vi "If Error, then NaN.vi"(5 "clear error (F)":bool, 6 "error in (T)":errorcluster={"status"=TRUE, "code"=-1, "source"="If Error, then NaN.vi"}, 7 "value3":dbl=3.0, 8 "value2":dbl=2.0, 9 "value1":dbl=1.0) -> (0 "error out":errorcluster, 1 "value out3":dbl=nan, 2 "value out2":dbl=nan, 3 "value out1":dbl=nan)   [LabVIEW 2020]
doc: "This function enables an error to be ignored, but marked with a NaN value in a double precision floating point variable.\n\nIf \"error in\" is TRUE, then \"value out\" is set to NaN, else \"value out\" is set to \"value in\".\n\nIf \"clear error\" is TRUE, then \"error out\" is set as follows: status is no error, code is 0, and source is an empty string."
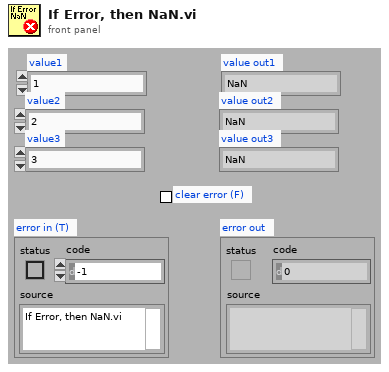
[diagram p1: front panel]
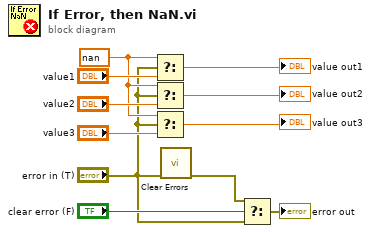
[diagram p0: block diagram]
diagram:
  w5 = nan ("NaN")
  n1 = Select(t=w5, s="error in (T)", f="value1") -> (s? t:f=→"value out1":dbl)
  n2 = Select(t=w5, s="error in (T)", f="value2") -> (s? t:f=→"value out2":dbl)
  n3 = Select(t=w5, s="error in (T)", f="value3") -> (s? t:f=→"value out3":dbl)
  n4 = call <vilib>:"Clear Errors.vi"("error in (no error)"="error in (T)") -> ("error out"=w3:errorcluster)  [unwired: 5 in, 1 out]
  n5 = Select(t=w3, s="clear error (F)", f="error in (T)") -> (s? t:f=→"error out":errorcluster)
